vi "GVSWait by Command Idx.vi"(11 "New Command Idx":i32) -> ()   [LabVIEW 2013]
uses:
  GVSNew View Global.vi
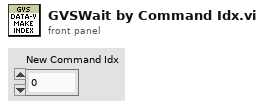
[diagram p1: front panel]
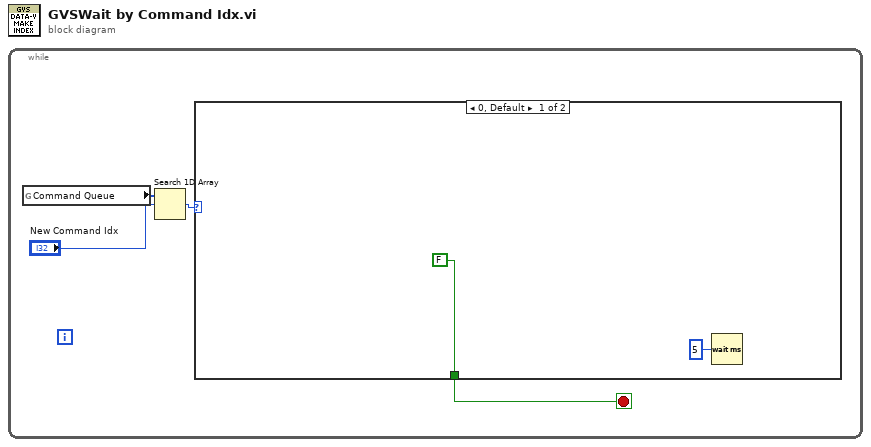
[diagram p0: block diagram]
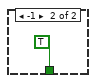
[diagram p2: hidden frame]
diagram:
  n1 = while {
    stop <- w2 stop-if-true
    n2 = global read "GVSNew View Global.vi" "Command Queue"() -> (w4:i32[])
    n3 = Search 1D Array(1D array=w4, element="New Command Idx") -> (index of element=w3:i32)  [unwired: 1 in]
    n4 = case shown="0, Default" w3 {
      tunnel: [FALSE TRUE] -> w2
      frame 0, Default {
        n5 = Wait (ms)(milliseconds to wait=u32 5) -> ()  [unwired: 1 out]
      }
      frame -1 {
      }
    }
  }
